vi "Hat Switch Interpreter.vi"(5 "POVs":i16[](array[numeric])) -> (0 "Buttons":bool[](array[boolean]), 1 "Buttons Pressed":bool[](array[boolean]), 2 "Enum Status":T2(ring), 3 "Numeric Status":u8, 4 "Hat Switch Cluster":T1)   [LabVIEW 2015]
panel:
  # "ENUM LAYOUT"
  # "NUMERIC LAYOUT"
  # "North"
  # "1"
  # "Northeast"
  # "2"
  # "Northwest"
  # "8"
  # "West"
  # "East"
  # "7"
  # "3"
  # "Null"
  # "0"
  # "Southwest"
  # "Southeast"
  # "6"
  # "4"
  # "5"
  # "South"
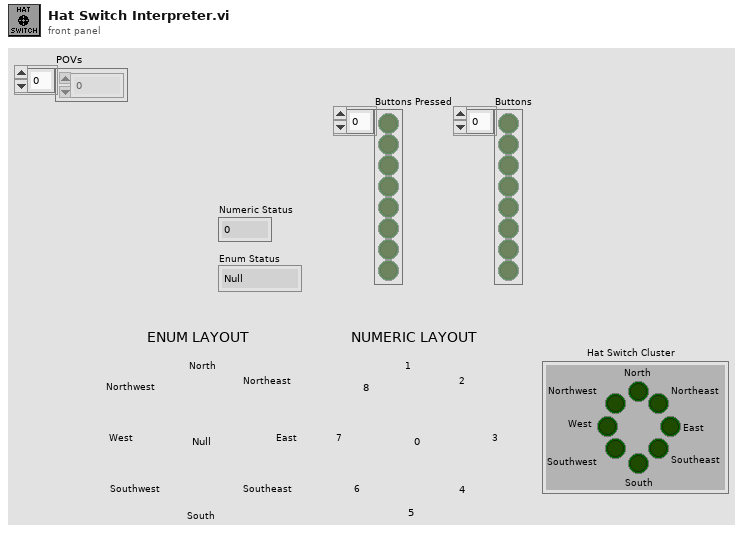
[diagram p1: front panel]
types:
  T1 = cluster{"North":bool, "Northeast":bool, "East":bool, "Southeast":bool, "South":bool, "Southwest":bool, "West":bool, "Northwest":bool}
  T2 = enum8{"Null", "North", "Northeast", "East", "Southeast", "South", "Southwest", "West", "Northwest"}
  T3 = cluster{"North":bool, "Northeast":bool, "East":bool, "Southeast":bool, "South":bool, "Northwest":bool, "Southwest":bool, "West":bool}
  T4 = cluster{"[0]":bool, "[1]":bool, "[2]":bool, "[3]":bool, "[4]":bool, "[5]":bool, "[6]":bool, "[7]":bool, "[8]":bool}
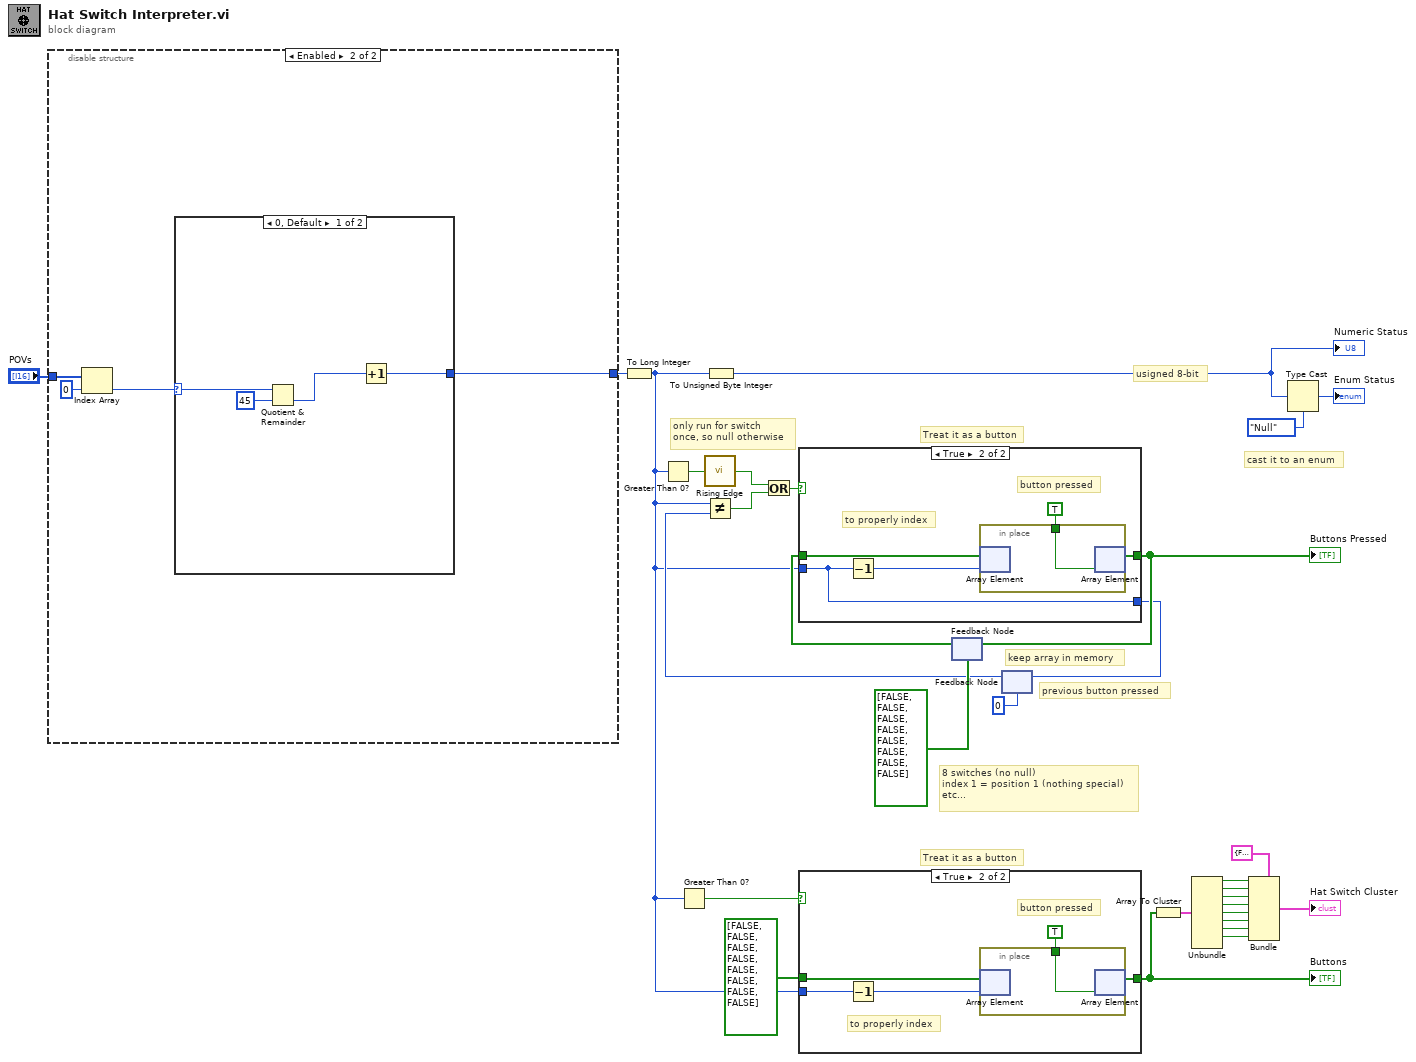
[diagram p0: block diagram]
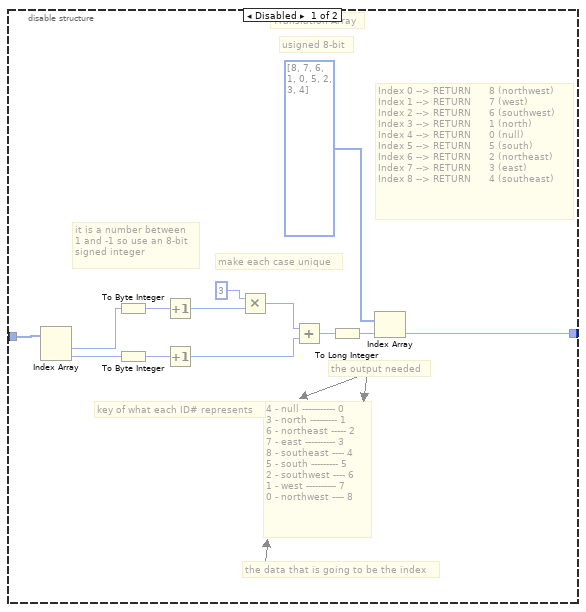
[diagram p2: hidden frame]
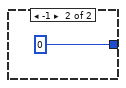
[diagram p3: hidden frame]
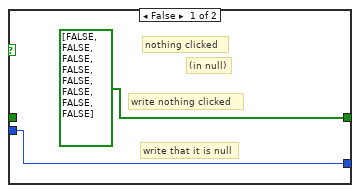
[diagram p5: hidden frame]
diagram:
  # "cast it to an enum"
  # "Treat it as a button"
  # "only run for switch\nonce, so null otherwise"
  # "keep array in memory"
  # "previous button pressed"
  # "8 switches (no null)\nindex 1 = position 1 (nothing special)\netc..."
  # "Treat it as a button"
  # "usigned 8-bit"
  n1 = disable-structure shown="Enabled" {
    disable-tunnel: [w34 w44] -> w22
    disable-tunnel: "POVs" -> [w33 w47]
    frame Disabled {
      # "usigned 8-bit"
      # "the data that is going to be the index"
      # "the output needed"
      # "key of what each ID# represents"
      # "Index 0 --> RETURN      8 (northwest)\nIndex 1 --> RETURN      7 (west)\nIndex 2 --> RETURN      6 (southwest)\nIndex 3 --> RETURN      1 (north)\nIndex 4 --> RETURN      0 (null)\nIndex 5 --> RETURN      5 (south)\nIndex 6 --> RETURN      2 (northeast)\nIndex 7 --> RETURN      3 (east)\nIndex 8 --> RETURN      4 (southeast)"
      # "4 - null ----------- 0\n3 - north --------- 1\n6 - northeast ----- 2\n7 - east ---------- 3\n8 - southeast ---- 4\n5 - south --------- 5\n2 - southwest ---- 6\n1 - west ---------- 7\n0 - northwest ---- 8"
      # "Translation Array"
      # "it is a number between\n1 and -1 so use an 8-bit\nsigned integer"
      # "make each case unique"
      n2 = Index Array(array=w33) -> (element #1=w32:i16, element #2=w31:i16)  [unwired: 2 in]
      n3 = To Byte Integer(number=w32) -> (8bit integer=w39:i8)
      n4 = To Byte Integer(number=w31) -> (8bit integer=w38:i8)
      n5 = Increment(x=w39) -> (x+1=w43:i8)
      n6 = Increment(x=w38) -> (x+1=w40:i8)
      n7 = Multiply(x=i8 3, y=w43) -> (x*y=w41:i8)
      n8 = Add(x=w41, y=w40) -> (x+y=w36:i8)
      n9 = To Long Integer(number=w36) -> (32bit integer=w35:i32)
      n10 = Index Array(array=u8[] [8, 7, 6, 1, 0, 5, 2, 3, 4], index=w35) -> (element=w34:u8)
    }
    frame Enabled {
      n11 = Index Array(array=w47, index=0) -> (element=w45:i16)
      n12 = case shown="0, Default" w45 {
        selector: w45 -> [w51 _]
        tunnel: [w48 i16 0] -> w44
        frame 0, Default {
          n13 = Quotient & Remainder(x=w51, y=i16 45) -> (floor(x/y)=w49:i16)  [unwired: 1 out]
          n14 = Increment(x=w49) -> (x+1=w48:i16)
        }
        frame -1 {
        }
      }
    }
  }
  n15 = To Long Integer(number=w22) -> (32bit integer=w19:i32)
  n16 = Greater Than 0?(x=w19) -> (x > 0?=w25:bool)
  n17 = Greater Than 0?(x=w19) -> (x > 0?=w2:bool)
  n18 = call "Rising Edge.vi"("Input"=w25) -> ("Rising Edge"=w24:bool)
  n19 = To Unsigned Byte Integer(number=w19) -> (unsigned 8bit integer=w6:u8)
  "Numeric Status" <- w6
  n20 = case shown="True" w2 {
    tunnel: [w53 w54] -> w18
    tunnel: w19 -> [_ w56]
    tunnel: bool[] [FALSE, FALSE, FALSE, FALSE, FALSE, FALSE, FALSE, FALSE] -> [w53 w55]
    frame False {
      # "write nothing clicked"
      # "(in null)"
      # "nothing clicked"
    }
    frame True {
      # "to properly index"
      # "button pressed"
      n21 = Decrement(x=w56) -> (x-1=w57:i32)
      n22 = in-place {
        in-place-border: TRUE -> [w59]
        n23 = in-place-array #1(w55, w57) -> ()  [unwired: 1 out]
        n24 = in-place-array #1(w59) -> (w54:bool[])  [unwired: 1 out]
      }
    }
  }
  "Buttons" <- w18
  n25 = feedback #2(bool[] [FALSE, FALSE, FALSE, FALSE, FALSE, FALSE, FALSE, FALSE]) -> (w29:bool[])
  n26 = feedback #3(0) -> (w20:i32)
  n27 = Not Equal?(x=w19, y=w20) -> (x != y?=w21:bool)
  n28 = Or(x=w24, y=w21) -> (x .or. y?=w23:bool)
  n29 = case shown="True" w23 {
    tunnel: w29 -> [_ w66]
    tunnel: [bool[] [FALSE, FALSE, FALSE, FALSE, FALSE, FALSE, FALSE, FALSE] w65] -> w28
    tunnel: w19 -> [w61 w62]
    tunnel: [w61 w62] -> w26
    frame False {
      # "write nothing clicked"
      # "write that it is null"
      # "(in null)"
      # "nothing clicked"
    }
    frame True {
      # "to properly index"
      # "button pressed"
      n30 = Decrement(x=w62) -> (x-1=w63:i32)
      n31 = in-place {
        in-place-border: TRUE -> [w67]
        n32 = in-place-array #4(w66, w63) -> ()  [unwired: 1 out]
        n33 = in-place-array #4(w67) -> (w65:bool[])  [unwired: 1 out]
      }
    }
  }
  "Buttons Pressed" <- w28
  n34 = feedback-in #2(w28) -> ()
  n35 = feedback-in #3(w26) -> ()
  n36 = Array To Cluster(array=w18) -> (cluster=w17:T4)
  n37 = Unbundle(w17) -> ("[0]"=w15:bool, "[1]"=w7:bool, "[2]"=w8:bool, "[3]"=w9:bool, "[4]"=w10:bool, "[5]"=w11:bool, "[6]"=w12:bool, "[7]"=w13:bool)  [unwired: 1 out]
  n38 = Bundle(cluster=T3 {"North"=FALSE, "Northeast"=FALSE, "East"=FALSE, "Southeast"=FALSE, "South"=FALSE, "Northwest"=FALSE, "Southwest"=FALSE, "West"=FALSE} ("Hat Switch Cluster"), "North"=w15, "Northeast"=w7, "East"=w8, "Southeast"=w9, "South"=w10, "Northwest"=w11, "Southwest"=w12, "West"=w13) -> (→"Hat Switch Cluster":T3)
  n39 = Type Cast(type=T2."Null" ("Enum Status"), x=w6) -> (*(type *) &x=→"Enum Status":T2)
